vi "Test Filter.vi"() -> ()   [LabVIEW 2021]
uses:
  Channels/ChannelRegistrar/typedef/Datatype CAN.ctl
  typedef/CAN Filter.ctl
  CAN_Logic.lvclass/CAN_Logic.ctl
  CAN_Logic.lvclass
  Channels/ChannelRegistrar/ChannelRegistrar.lvlib
panel:
  in  "Filter":T1={"Allow List (ID)"=[], "Deny List (ID)"=[120, 2]} {"Deny List (ID)" format="%.0x"; "Allow List (ID)" format="%.0x"}
  out "CAN Data out":T2[](array[typedef])=[{"payload"=[], "identifier"=1, "Tags"=0, "Timestamp"=0}, {"payload"=[], "identifier"=222599, "Tags"=0, "Timestamp"=0}] {"Tags" format="%.0x"; "payload" format="%x"; "identifier" format="%x"}
  in  "CAN Data in":T2[](array[typedef])=[{"payload"=[], "identifier"=1, "Tags"=0, "Timestamp"=0}, {"payload"=[], "identifier"=2, "Tags"=0, "Timestamp"=0}, {"payload"=[], "identifier"=222599, "Tags"=0, "Timestamp"=0}, {"payload"=[], "identifier"=120, "Tags"=0, "Timestamp"=0}] {"Tags" format="%.0x"; "payload" format="%x"; "identifier" format="%x"}
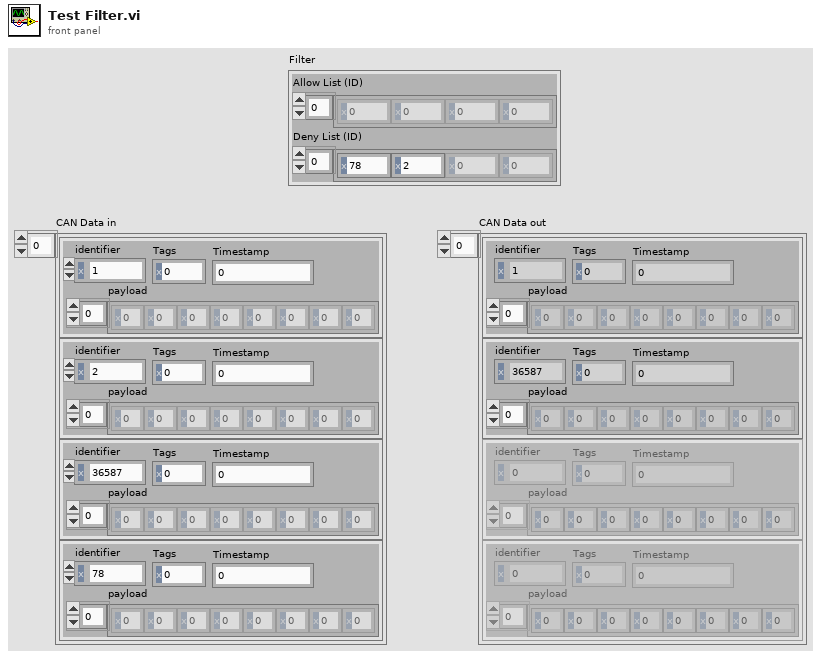
[diagram p1: front panel]
types:
  T1 = typedef "CAN_Logic.lvclass/CAN Filter.ctl" = cluster{"Allow List (ID)":u32[], "Deny List (ID)":u32[]}
  T2 = typedef "ChannelRegistrar.lvlib/Datatype CAN.ctl" = cluster{"payload":u8[], "identifier":u32, "Tags":u8, "Timestamp":u64}
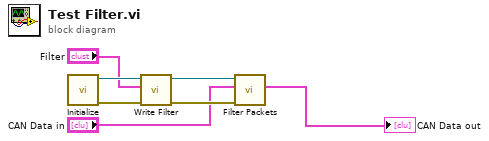
[diagram p0: block diagram]
diagram:
  n1 = call "Initialize.vi"() -> ("error out"=w6:errorcluster, "CAN_Logic out"=w7:refnum<class "CAN_Logic.lvclass">)  [unwired: 10 in]
  n2 = call "Write Filter.vi"("error in (no error)"=w6, "Filter"="Filter", "CAN_Logic in"=w7) -> ("error out"=w3:errorcluster, "CAN_Logic out"=w4:refnum<class "CAN_Logic.lvclass">)  [unwired: 7 in]
  n3 = call "Filter Packets.vi"("error in (no error)"=w3, "CAN Data in"="CAN Data in", "CAN_Logic in"=w4) -> ("CAN Data out"=→"CAN Data out":T2[])  [unwired: 6 in, 2 out]
